vi "TGC&RF_ADInfo.vi"(0 "refnum":refnum<file>, 11 "offset":i32) -> (2 "TGC & RF/AD Info":T1, 4 "dup refnum":refnum<file>, 6 "avg num":i16, 8 "filler":string, 10 "c speed":i16, 15 "DivideBy":i16)   [LabVIEW 2022 SP3]
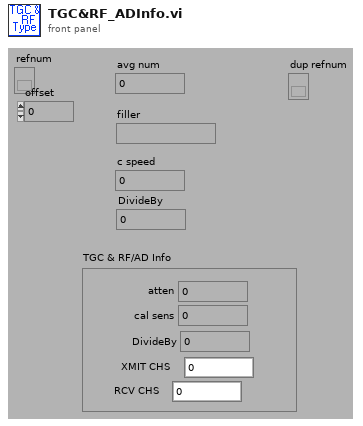
[diagram p1: front panel]
types:
  T1 = cluster{"atten":i16, "cal sens":i16, "DivideBy":i16, "XMIT CHS":u8, "RCV CHS":u8}
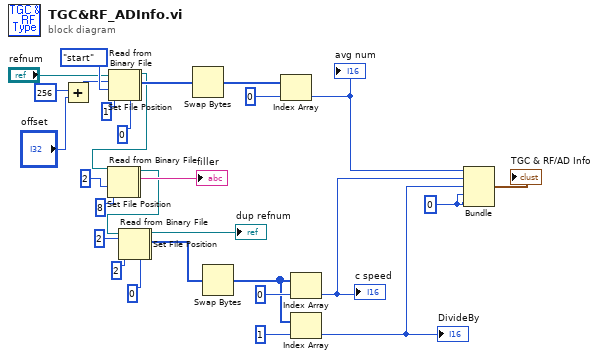
[diagram p0: block diagram]
diagram:
  w1 = u8 0
  n1 = Add(x=256 ("pos offset (0)"), y="offset") -> (x+y=w10:i32)
  n2 = Set File Position(offset (in bytes) (0)=w10, refnum="refnum", from (0:start)=enum16{"start", "end", "current"}."start" ("pos mode (0:2)")) -> (refnum out=w5:refnum<file>, error out=w4:errorcluster)  [unwired: 1 in]
  n3 = Read from Binary File(5:i16 0, 8:w4, 10:1 ("count"), 11:w5) -> (2:w28:i16[], 3:w26:refnum<file>)  [unwired: 4 out]
  n4 = Set File Position(refnum=w26, from (0:start)=2) -> (refnum out=w3:refnum<file>, error out=w2:errorcluster)  [unwired: 1 in, 1 out]
  n5 = Read from Binary File(8:w2, 10:8 ("count"), 11:w3) -> (2:→"filler":string, 3:w16:refnum<file>)  [unwired: 5 out]
  n6 = Set File Position(refnum=w16, from (0:start)=2) -> (refnum out=w7:refnum<file>, error out=w6:errorcluster)  [unwired: 1 in, 1 out]
  n7 = Read from Binary File(5:i16 0, 8:w6, 10:2 ("count"), 11:w7) -> (2:w20:i16[], 3:→"dup refnum":refnum<file>)  [unwired: 4 out]
  n8 = Swap Bytes(anything=w28) -> (byte swapped=w18:i16[])
  n9 = Swap Bytes(anything=w20) -> (byte swapped=w19:i16[])
  n10 = Index Array(array=w18, index=0) -> (element=w14:i16)
  "avg num" <- w14
  n11 = Index Array(array=w19, index=0) -> (element=w13:i16)
  "c speed" <- w13
  n12 = Index Array(array=w19, index=1) -> (element=w12:i16)
  "DivideBy" <- w12
  n13 = Bundle(w14, w13, w12, w1, w1) -> (→"TGC & RF/AD Info":cluster{i16, i16, i16, u8, u8})  [unwired: 1 out]
